vi "Weather Parse Test.vi"() -> ()   [LabVIEW 2020, in "CDM-Config.lvlib"] (continued)
,\n                    \"UGC\": [\n                        \"PKZ773\"\n                    ]\n                },\n                \"affectedZones\": [\n                    \"https://api.weather.gov/zones/forecast/PKZ773\"\n                ],\n                \"references\": [],\n                \"sent\": \"2025-12-02T16:08:00-09:00\",\n                \"effective\": \"2025-12-02T16:08:00-09:00\",\n                \"onset\": \"2025-12-03T05:00:00-09:00\",\n                \"expires\": \"2025-12-03T05:15:00-09:00\",\n                \"ends\": \"2025-12-04T05:00:00-09:00\",\n                \"status\": \"Actual\",\n                \"messageType\": \"Alert\",\n                \"category\": \"Met\",\n                \"severity\": \"Minor\",\n                \"certainty\": \"Likely\",\n                \"urgency\": \"Expected\",\n                \"event\": \"Small Craft Advisory\",\n                \"sender\": \"w-nws.webmaster@noaa.gov\",\n                \"senderName\": \"NWS Anchorage AK\",\n                \"headline\": \"Small Craft Advisory issued December 2 at 4:08PM AKST until December 4 at 5:00AM AKST by NWS Anchorage AK\",\n                \"description\": \"Coastal Waters Forecast for Southwest Alaska+Bristol Bay+The\\nAlaska Peninsula Waters and the Aleutian Islands up to 100 nm out.\\n\\nWind forecasts reflect the predominant speed and direction\\nexpected. Sea forecasts represent an average of the highest\\none-third of the combined wind wave and swell height.\\n\\n.TONIGHT...SE wind 30 kt. Seas 18 ft. Rain.\\n.WED...NE wind 25 kt. Seas 15 ft. Rain.\\n.WED NIGHT...N wind 20 kt. Seas 10 ft.\\n.THU AND THU NIGHT...NE wind 15 kt. Seas 7 ft.\\n.FRI...NE wind 25 kt. Seas 5 ft.\\n.SAT THROUGH SUN...N wind 30 kt. Seas 7 ft.\",\n                \"instruction\": null,\n                \"response\": \"Avoid\",\n                \"parameters\": {\n                    \"AWIPSidentifier\": [\n                        \"CWFALU\"\n                    ],\n                    \"WMOidentifier\": [\n                        \"FZAK52 PAFC 030108\"\n                    ],\n                    \"NWSheadline\": [\n                        \"SMALL CRAFT ADVISORY THROUGH WEDNESDAY NIGHT\"\n                    ],\n                    \"BLOCKCHANNEL\": [\n                        \"EAS\",\n                        \"NWEM\",\n                        \"CMAS\"\n                    ],\n                    \"VTEC\": [\n                        \"/O.NEW.PAFC.SC.Y.9907.251203T1400Z-251204T1400Z/\"\n                    ],\n                    \"eventEndingTime\": [\n                        \"2025-12-04T05:00:00-09:00\"\n                    ]\n                },\n                \"scope\": \"Public\",\n                \"code\": \"IPAWSv1.0\",\n                \"language\": \"en-US\",\n                \"web\": \"http://www.weather.gov\",\n                \"eventCode\": {\n                    \"SAME\": [\n                        \"NWS\"\n                    ],\n                    \"NationalWeatherService\": [\n                        \"SCY\"\n                    ]\n                }\n            }\n        },\n        {\n            \"id\": \"https://api.weather.gov/alerts/urn:oid:2.49.0.1.840.0.90d765b84bbb08e28d74a226f4e1f9e6e65de885.013.1\",\n            \"type\": \"Feature\",\n            \"geometry\": null,\n            \"properties\": {\n                \"@id\": \"https://api.weather.gov/alerts/urn:oid:2.49.0.1.840.0.90d765b84bbb08e28d74a226f4e1f9e6e65de885.013.1\",\n                \"@type\": \"wx:Alert\",\n                \"id\": \"urn:oid:2.49.0.1.840.0.90d765b84bbb08e28d74a226f4e1f9e6e65de885.013.1\",\n                \"areaDesc\": \"Cape Sarichef to Nikoski Bering Side from 15 to 85 NM\",\n                \"geocode\": {\n                    \"SAME\": [\n                        \"058772\"\n                    ],\n                    \"UGC\": [\n                        \"PKZ772\"\n                    ]\n                },\n                \"affectedZones\": [\n                    \"https://api.weather.gov/zones/forecast/PKZ772\"\n                ],\n                \"references\": [],\n                \"sent\": \"2025-12-02T16:08:00-09:00\",\n                \"effective\": \"2025-12-02T16:08:00-09:00\",\n                \"onset\": \"2025-12-03T05:00:00-09:00\",\n                \"expires\": \"2025-12-03T05:15:00-09:00\",\n                \"ends\": \"2025-12-04T05:00:00-09:00\",\n                \"status\": \"Actual\",\n                \"messageType\": \"Alert\",\n                \"category\": \"Met\",\n                \"severity\": \"Minor\",\n                \"certainty\": \"Likely\",\n                \"urgency\": \"Expected\",\n                \"event\": \"Small Craft Advisory\",\n                \"sender\": \"w-nws.webmaster@noaa.gov\",\n                \"senderName\": \"NWS Anchorage AK\",\n                \"headline\": \"Small Craft Advisory issued December 2 at 4:08PM AKST until December 4 at 5:00AM AKST by NWS Anchorage AK\",\n                \"description\": \"Coastal Waters Forecast for Southwest Alaska+Bristol Bay+The\\nAlaska Peninsula Waters and the Aleutian Islands up to 100 nm out.\\n\\nWind forecasts reflect the predominant speed and direction\\nexpected. Sea forecasts represent an average of the highest\\none-third of the combined wind wave and swell height.\\n\\n.TONIGHT...E wind 30 kt. Seas 18 ft. Rain.\\n.WED...NE wind 30 kt. Seas 15 ft. Rain.\\n.WED NIGHT...N wind 30 kt. Seas 16 ft.\\n.THU...NE wind 30 kt. Seas 14 ft.\\n.THU NIGHT...NE wind 25 kt. Seas 10 ft.\\n.FRI...NE wind 25 kt. Seas 7 ft.\\n.SAT...N wind 30 kt. Seas 15 ft.\\n.SUN...N wind 40 kt. Seas 21 ft.\",\n                \"instruction\": null,\n                \"response\": \"Avoid\",\n                \"parameters\": {\n                    \"AWIPSidentifier\": [\n                        \"CWFALU\"\n                    ],\n                    \"WMOidentifier\": [\n                        \"FZAK52 PAFC 030108\"\n                    ],\n                    \"NWSheadline\": [\n                        \"SMALL CRAFT ADVISORY THROUGH WEDNESDAY NIGHT\"\n                    ],\n                    \"BLOCKCHANNEL\": [\n                        \"EAS\",\n                        \"NWEM\",\n                        \"CMAS\"\n                    ],\n                    \"VTEC\": [\n                        \"/O.NEW.PAFC.SC.Y.9905.251203T1400Z-251204T1400Z/\"\n                    ],\n                    \"eventEndingTime\": [\n                        \"2025-12-04T05:00:00-09:00\"\n                    ]\n                },\n                \"scope\": \"Public\",\n                \"code\": \"IPAWSv1.0\",\n                \"language\": \"en-US\",\n                \"web\": \"http://www.weather.gov\",\n                \"eventCode\": {\n                    \"SAME\": [\n                        \"NWS\"\n                    ],\n                    \"NationalWeatherService\": [\n                        \"SCY\"\n                    ]\n                }\n            }\n        },\n        {\n            \"id\": \"https://api.weather.gov/alerts/urn:oid:2.49.0.1.840.0.90d765b84bbb08e28d74a226f4e1f9e6e65de885.012.1\",\n            \"type\": \"Feature\",\n            \"geometry\": null,\n            \"properties\": {\n                \"@id\": \"https://api.weather.gov/alerts/urn:oid:2.49.0.1.840.0.90d765b84bbb08e28d74a226f4e1f9e6e65de885.012.1\",\n                \"@type\": \"wx:Alert\",\n                \"id\": \"urn:oid:2.49.0.1.840.0.90d765b84bbb08e28d74a226f4e1f9e6e65de885.012.1\",\n                \"areaDesc\": \"Cape Sarichef to Nikoski Bering Side out to 15 NM\",\n                \"geocode\": {\n                    \"SAME\": [\n                        \"058770\"\n                    ],\n                    \"UGC\": [\n                        \"PKZ770\"\n                    ]\n                },\n                \"affectedZones\": [\n                    \"https://api.weather.gov/zones/forecast/PKZ770\"\n                ],\n                \"references\": [],\n                \"sent\": \"2025-12-02T16:08:00-09:00\",\n                \"effective\": \"2025-12-02T16:08:00-09:00\",\n                \"onset\": \"2025-12-03T05:00:00-09:00\",\n                \"expires\": \"2025-12-03T05:15:00-09:00\",\n                \"ends\": \"2025-12-04T05:00:00-09:00\",\n                \"status\": \"Actual\",\n                \"messageType\": \"Alert\",\n                \"category\": \"Met\",\n                \"severity\": \"Minor\",\n                \"certainty\": \"Likely\",\n                \"urgency\": \"Expected\",\n                \"event\": \"Small Craft Advisory\",\n                \"sender\": \"w-nws.webmaster@noaa.gov\",\n                \"senderName\": \"NWS Anchorage AK\",\n                \"headline\": \"Small Craft Advisory issued December 2 at 4:08PM AKST until December 4 at 5:00AM AKST by NWS Anchorage AK\",\n                \"description\": \"Coastal Waters Forecast for Southwest Alaska+Bristol Bay+The\\nAlaska Peninsula Waters and the Aleutian Islands up to 100 nm out.\\n\\nWind forecasts reflect the predominant speed and direction\\nexpected. Sea forecasts represent an average of the highest\\none-third of the combined wind wave and swell height.\\n\\n.TONIGHT...E wind 30 kt. Seas 16 ft. Rain.\\n.WED...NE wind 30 kt. Seas 13 ft. Rain.\\n.WED NIGHT...N wind 30 kt. Seas 14 ft. Rain.\\n.THU...NE wind 25 kt. Seas 13 ft.\\n.THU NIGHT...E wind 20 kt. Seas 9 ft.\\n.FRI...E wind 20 kt. Seas 6 ft.\\n.SAT...N wind 30 kt. Seas 14 ft.\\n.SUN...N wind 35 kt. Seas 18 ft.\",\n                \"instruction\": null,\n                \"response\": \"Avoid\",\n                \"parameters\": {\n                    \"AWIPSidentifier\": [\n                        \"CWFALU\"\n                    ],\n                    \"WMOidentifier\": [\n                        \"FZAK52 PAFC 030108\"\n                    ],\n                    \"NWSheadline\": [\n                        \"SMALL CRAFT ADVISORY THROUGH WEDNESDAY NIGHT\"\n                    ],\n                    \"BLOCKCHANNEL\": [\n                        \"EAS\",\n                        \"NWEM\",\n                        \"CMAS\"\n                    ],\n                    \"VTEC\": [\n                        \"/O.NEW.PAFC.SC.Y.9904.251203T1400Z-251204T1400Z/\"\n                    ],\n                    \"eventEndingTime\": [\n                        \"2025-12-04T05:00:00-09:00\"\n                    ]\n                },\n                \"scope\": \"Public\",\n                \"code\": \"IPAWSv1.0\",\n                \"language\": \"en-US\",\n                \"web\": \"http://www.weather.gov\",\n                \"eventCode\": {\n                    \"SAME\": [\n                        \"NWS\"\n                    ],\n                    \"NationalWeatherService\": [\n                        \"SCY\"\n                    ]\n                }\n            }\n        },\n        {\n            \"id\": \"https://api.weather.gov/alerts/urn:oid:2.49.0.1.840.0.90d765b84bbb08e28d74a226f4e1f9e6e65de885.018.1\",\n            \"type\": \"Feature\",\n            \"geometry\": null,\n            \"properties\": {\n                \"@id\": \"https://api.weather.gov/alerts/urn:oid:2.49.0.1.840.0.90d765b84bbb08e28d74a226f4e1f9e6e65de885.018.1\",\n                \"@type\": \"wx:Alert\",\n                \"id\": \"urn:oid:2.49.0.1.840.0.90d765b84bbb08e28d74a226f4e1f9e6e65de885.018.1\",\n                \"areaDesc\": \"Nikolski to Seguam Bering Side from 15 to 85 NM\",\n                \"geocode\": {\n                    \"SAME\": [\n                        \"058776\"\n                    ],\n                    \"UGC\": [\n                        \"PKZ776\"\n                    ]\n                },\n                \"affectedZones\": [\n                    \"https://api.weather.gov/zones/forecast/PKZ776\"\n                ],\n                \"references\": [],\n                \"sent\": \"2025-12-02T16:08:00-09:00\",\n                \"effective\": \"2025-12-02T16:08:00-09:00\",\n                \"onset\": \"2025-12-03T05:00:00-09:00\",\n                \"expires\": \"2025-12-03T05:15:00-09:00\",\n                \"ends\": \"2025-12-04T05:00:00-09:00\",\n                \"status\": \"Actual\",\n                \"messageType\": \"Alert\",\n                \"category\": \"Met\",\n                \"severity\": \"Moderate\",\n                \"certainty\": \"Likely\",\n                \"urgency\": \"Expected\",\n                \"event\": \"Gale Warning\",\n                \"sender\": \"w-nws.webmaster@noaa.gov\",\n                \"senderName\": \"NWS Anchorage AK\",\n                \"headline\": \"Gale Warning issued December 2 at 4:08PM AKST until December 4 at 5:00AM AKST by NWS Anchorage AK\",\n                \"description\": \"Coastal Waters Forecast for Southwest Alaska+Bristol Bay+The\\nAlaska Peninsula Waters and the Aleutian Islands up to 100 nm out.\\n\\nWind forecasts reflect the predominant speed and direction\\nexpected. Sea forecasts represent an average of the highest\\none-third of the combined wind wave and swell height.\\n\\n.TONIGHT...N wind 45 kt diminishing to 35 kt after midnight. Seas\\n31 ft. Rain.\\n.WED...N wind 35 kt. Seas 23 ft. Rain.\\n.WED NIGHT...N wind 35 kt. Seas 20 ft.\\n.THU...N wind 30 kt. Seas 15 ft.\\n.THU NIGHT...NE wind 20 kt. Seas 10 ft.\\n.FRI...E wind 15 kt. Seas 8 ft.\\n.SAT...N wind 30 kt. Seas 12 ft.\\n.SUN...N wind 40 kt. Seas 22 ft.\",\n                \"instruction\": null,\n                \"response\": \"Avoid\",\n                \"parameters\": {\n                    \"AWIPSidentifier\": [\n                        \"CWFALU\"\n                    ],\n                    \"WMOidentifier\": [\n                        \"FZAK52 PAFC 030108\"\n                    ],\n                    \"NWSheadline\": [\n                        \"GALE WARNING THROUGH WEDNESDAY NIGHT\"\n                    ],\n                    \"BLOCKCHANNEL\": [\n                        \"EAS\",\n                        \"NWEM\",\n                        \"CMAS\"\n                    ],\n                    \"VTEC\": [\n                        \"/O.NEW.PAFC.GL.W.9910.251203T1400Z-251204T1400Z/\"\n                    ],\n                    \"eventEndingTime\": [\n                        \"2025-12-04T05:00:00-09:00\"\n                    ]\n                },\n                \"scope\": \"Public\",\n                \"code\": \"IPAWSv1.0\",\n                \"language\": \"en-US\",\n                \"web\": \"http://www.weather.gov\",\n                \"eventCode\": {\n                    \"SAME\": [\n                        \"NWS\"\n                    ],\n                    \"NationalWeatherService\": [\n                        \"GLW\"\n                    ]\n                }\n            }\n        },\n        {\n            \"id\": \"https://api.weather.gov/alerts/urn:oid:2.49.0.1.840.0.90d765b84bbb08e28d74a226f4e1f9e6e65de885.004.1\",\n            \"type\": \"Feature\",\n            \"geometry\": null,\n            \"properties\": {\n                \"@id\": \"https://api.weather.gov/alerts/urn:oid:2.49.0.1.840.0.90d765b84bbb08e28d74a226f4e1f9e6e65de885.004.1\",\n                \"@type\": \"wx:Alert\",\n                \"id\": \"urn:oid:2.49.0.1.840.0.90d765b84bbb08e28d74a226f4e1f9e6e65de885.004.1\",\n                \"areaDesc\": \"Castle Cape to Cape Tolstoi out to 15 NM\",\n                \"geocode\": {\n                    \"SAME\": [\n                        \"058752\"\n                    ],\n                    \"UGC\": [\n                        \"PKZ752\"\n                    ]\n                },\n                \"affectedZones\": [\n                    \"https://api.weather.gov/zones/forecast/PKZ752\"\n                ],\n                \"references\": [],\n                \"sent\": \"2025-12-02T16:08:00-09:00\",\n                \"effective\": \"2025-12-02T16:08:00-09:00\",\n                \"onset\": \"2025-12-03T05:00:00-09:00\",\n                \"expires\": \"2025-12-03T05:15:00-09:00\",\n                \"ends\": \"2025-12-04T05:00:00-09:00\",\n                \"status\": \"Actual\",\n                \"messageType\": \"Alert\",\n                \"category\": \"Met\",\n                \"severity\": \"Minor\",\n                \"certainty\": \"Likely\",\n                \"urgency\": \"Expected\",\n                \"event\": \"Small Craft Advisory\",\n                \"sender\": \"w-nws.webmaster@noaa.gov\",\n                \"senderName\": \"NWS Anchorage AK\",\n                \"headline\": \"Small Craft Advisory issued December 2 at 4:08PM AKST until December 4 at 5:00AM AKST by NWS Anchorage AK\",\n                \"description\": \"Coastal Waters Forecast for Southwest Alaska+Bristol Bay+The\\nAlaska Peninsula Waters and the Aleutian Islands up to 100 nm out.\\n\\nWind forecasts reflect the predominant speed and direction\\nexpected. Sea forecasts represent an average of the highest\\none-third of the combined wind wave and swell height.\\n\\n.TONIGHT...SE wind 25 kt. Seas 13 ft. Rain.\\n.WED...SE wind 20 kt. Seas 10 ft. Rain.\\n.WED NIGHT...SE wind 20 kt. Seas 10 ft. Rain.\\n.THU...E wind 20 kt. Seas 8 ft.\\n.THU NIGHT...NE wind 25 kt. Seas 8 ft.\\n.FRI...N wind 20 kt. Seas 8 ft.\\n.SAT...NW wind 35 kt. Seas 5 ft.\\n.SUN...N wind 20 kt. Seas 2 ft.\",\n                \"instruction\": null,\n                \"response\": \"Avoid\",\n                \"parameters\": {\n                    \"AWIPSidentifier\": [\n                        \"CWFALU\"\n                    ],\n                    \"WMOidentifier\": [\n                        \"FZAK52 PAFC 030108\"\n                    ],\n                    \"NWSheadline\": [\n                        \"SMALL CRAFT ADVISORY THROUGH WEDNESDAY NIGHT\"\n                    ],\n                    \"BLOCKCHANNEL\": [\n                        \"EAS\",\n                        \"NWEM\",\n                        \"CMAS\"\n                    ],\n                    \"VTEC\": [\n                        \"/O.NEW.PAFC.SC.Y.9896.251203T1400Z-251204T1400Z/\"\n                    ],\n                    \"eventEndingTime\": [\n                        \"2025-12-04T05:00:00-09:00\"\n                    ]\n                },\n                \"scope\": \"Public\",\n                \"code\": \"IPAWSv1.0\",\n                \"language\": \"en-US\",\n                \"web\": \"http://www.weather.gov\",\n                \"eventCode\": {\n                    \"SAME\": [\n                        \"NWS\"\n                    ],\n                    \"NationalWeatherService\": [\n                        \"SCY\"\n                    ]\n                }\n            }\n        },\n        {\n            \"id\": \"https://api.weather.gov/alerts/urn:oid:2.49.0.1.840.0.90d765b84bbb08e28d74a226f4e1f9e6e65de885.005.1\",\n            \"type\": \"Feature\",\n            \"geometry\": null,\n            \"properties\": {\n                \"@id\": \"https://api.weather.gov/alerts/urn:oid:2.49.0.1.840.0.90d765b84bbb08e28d74a226f4e1f9e6e65de885.005.1\",\n                \"@type\": \"wx:Alert\",\n                \"id\": \"urn:oid:2.49.0.1.840.0.90d765b84bbb08e28d74a226f4e1f9e6e65de885.005.1\",\n                \"areaDesc\": \"Castle Cape to Cape Tolstoi from 15 to 100 NM\",\n                \"geocode\": {\n                    \"SAME\": [\n                        \"058753\"\n                    ],\n                    \"UGC\": [\n                        \"PKZ753\"\n                    ]\n                },\n                \"affectedZones\": [\n                    \"https://api.weather.gov/zones/forecast/PKZ753\"\n                ],\n                \"references\": [],\n                \"sent\": \"2025-12-02T16:08:00-09:00\",\n                \"effective\": \"2025-12-02T16:08:00-09:00\",\n                \"onset\": \"2025-12-03T05:00:00-09:00\",\n                \"expires\": \"2025-12-03T05:15:00-09:00\",\n                \"ends\": \"2025-12-04T05:00:00-09:00\",\n                \"status\": \"Actual\",\n                \"messageType\": \"Alert\",\n                \"category\": \"Met\",\n                \"severity\": \"Minor\",\n                \"certainty\": \"Likely\",\n                \"urgency\": \"Expected\",\n                \"event\": \"Small Craft Advisory\",\n                \"sender\": \"w-nws.webmaster@noaa.gov\",\n                \"senderName\": \"NWS Anchorage AK\",\n                \"headline\": \"Small Craft Advisory issued December 2 at 4:08PM AKST until December 4 at 5:00AM AKST by NWS Anchorage AK\",\n                \"description\": \"Coastal Waters Forecast for Southwest Alaska+Bristol Bay+The\\nAlaska Peninsula Waters and the Aleutian Islands up to 100 nm out.\\n\\nWind forecasts reflect the predominant speed and direction\\nexpected. Sea forecasts represent an average of the highest\\none-third of the combined wind wave and swell height.\\n\\n.TONIGHT...SE wind 30 kt. Seas 19 ft.\\n.WED...S wind 25 kt. Seas 17 ft. Rain.\\n.WED NIGHT...S wind 20 kt. Seas 16 ft. Rain.\\n.THU...E wind 20 kt. Seas 12 ft.\\n.THU NIGHT...NE wind 30 kt. Seas 9 ft.\\n.FRI...NW wind 20 kt. Seas 9 ft.\\n.SAT...NW wind 35 kt. Seas 13 ft.\\n.SUN...N wind 25 kt. Seas 11 ft.\",\n                \"instruction\": null,\n                \"response\": \"Avoid\",\n                \"parameters\": {\n                    \"AWIPSidentifier\": [\n                        \"CWFALU\"\n                    ],\n                    \"WMOidentifier\": [\n                        \"FZAK52 PAFC 030108\"\n                    ],\n                    \"NWSheadline\": [\n                        \"SMALL CRAFT ADVISORY THROUGH WEDNESDAY NIGHT\"\n                    ],\n                    \"BLOCKCHANNEL\": [\n                        \"EAS\",\n                        \"NWEM\",\n                        \"CMAS\"\n                    ],\n                    \"VTEC\": [\n                        \"/O.NEW.PAFC.SC.Y.9897.251203T1400Z-251204T1400Z/\"\n                    ],\n                    \"eventEndingTime\": [\n                        \"2025-12-04T05:00:00-09:00\"\n                    ]\n                },\n                \"scope\": \"Public\",\n                \"code\": \"IPAWSv1.0\",\n                \"language\": \"en-US\",\n                \"web\": \"http://www.weather.gov\",\n                \"eventCode\": {\n                    \"SAME\": [\n                        \"NWS\"\n                    ],\n                    \"NationalWeatherService\": [\n                        \"SCY\"\n                    ]\n                }\n            }\n        },\n        {\n            \"id\": \"https://api.weather.gov/alerts/urn:oid:2.49.0.1.840.0.90d765b84bbb08e28d74a226f4e1f9e6e65de885.023.1\",\n            \"type\": \"Feature\",\n            \"geometry\": null,\n            \"properties\": {\n                \"@id\": \"https://api.weather.gov/alerts/urn:oid:2.49.0.1.840.0.90d765b84bbb08e28d74a226f4e1f9e6e65de885.023.1\",\n                \"@type\": \"wx:Alert\",\n                \"id\": \"urn:oid:2.49.0.1.840.0.90d765b84bbb08e28d74a226f4e1f9e6e65de885.023.1\",\n                \"areaDesc\": \"Seguam to Adak Pacific Side out to 15 NM\",\n                \"geocode\": {\n                    \"SAME\": [\n                        \"058782\"\n                    ],\n                    \"UGC\": [\n                        \"PKZ782\"\n                    ]\n                },\n                \"affectedZones\": [\n                    \"https://api.weather.gov/zones/forecast/PKZ782\"\n                ],\n                \"references\": [],\n                \"sent\": \"2025-12-02T16:08:00-09:00\",\n                \"effective\": \"2025-12-02T16:08:00-09:00\",\n                \"onset\": \"2025-12-02T16:00:00-09:00\",\n                \"expires\": \"2025-12-03T05:15:00-09:00\",\n                \"ends\": \"2025-12-03T17:00:00-09:00\",\n                \"status\": \"Actual\",\n                \"messageType\": \"Alert\",\n                \"category\": \"Met\",\n                \"severity\": \"Moderate\",\n                \"certainty\": \"Likely\",\n                \"urgency\": \"Expected\",\n                \"event\": \"Gale Warning\",\n                \"sender\": \"w-nws.webmaster@noaa.gov\",\n                \"senderName\": \"NWS Anchorage AK\",\n                \"headline\": \"Gale Warning issued December 2 at 4:08PM AKST until December 3 at 5:00PM AKST by NWS Anchorage AK\",\n                \"description\": \"Coastal Waters Forecast for Southwest Alaska+Bristol Bay+The\\nAlaska Peninsula Waters and the Aleutian Islands up to 100 nm out.\\n\\nWind forecasts reflect the predominant speed and direction\\nexpected. Sea forecasts represent an average of the highest\\none-third of the combined wind wave and swell height.\\n\\n.TONIGHT...N wind 45 kt. Seas 15 ft. Rain.\\n.WED...N wind 35 kt. Seas 14 ft. Rain.\\n.WED NIGHT...N wind 30 kt. Seas 11 ft.\\n.THU...N wind 30 kt. Seas 8 ft.\\n.THU NIGHT...NE wind 15 kt. Seas 5 ft.\\n.FRI...NE wind 15 kt. Seas 10 ft.\\n.SAT...NE wind 25 kt. Seas 10 ft.\\n.SUN...N wind 35 kt. Seas 12 ft.\",\n                \"instruction\": null,\n                \"response\": \"Avoid\",\n                \"parameters\": {\n                    \"AWIPSidentifier\": [\n                        \"CWFALU\"\n                    ],\n                    \"WMOidentifier\": [\n                        \"FZAK52 PAFC 030108\"\n                    ],\n                    \"NWSheadline\": [\n                        \"GALE WARNING THROUGH WEDNESDAY\"\n                    ],\n                    \"BLOCKCHANNEL\": [\n                        \"EAS\",\n                        \"NWEM\",\n                        \"CMAS\"\n                    ],\n                    \"VTEC\": [\n                        \"/O.NEW.PAFC.GL.W.9915.251203T0100Z-251204T0200Z/\"\n                    ],\n                    \"eventEndingTime\": [\n                        \"2025-12-03T17:00:00-09:00\"\n                    ]\n                },\n                \"scope\": \"Public\",\n                \"code\": \"IPAWSv1.0\",\n                \"language\": \"en-US\",\n                \"web\": \"http://www.weather.gov\",\n                \"eventCode\": {\n                    \"SAME\": [\n                        \"NWS\"\n                    ],\n                    \"NationalWeatherService\": [\n                        \"GLW\"\n                    ]\n                }\n            }\n        },\n        {\n            \"id\": \"https://api.weather.gov/alerts/urn:oid:2.49.0.1.840.0.90d765b84bbb08e28d74a226f4e1f9e6e65de885.026.1\",\n            \"type\": \"Feature\",\n            \"geometry\": null,\n            \"properties\": {\n                \"@id\": \"https://api.weather.gov/alerts/urn:oid:2.49.0.1.840.0.90d765b84bbb08e28d74a226f4e1f9e6e65de885.026.1\",\n                \"@type\": \"wx:Alert\",\n                \"id\": \"urn:oid:2.49.0.1.840.0.90d765b84bbb08e28d74a226f4e1f9e6e65de885.026.1\",\n                \"areaDesc\": \"Adak to Kiska Pacific Side\",\n                \"geocode\": {\n                    \"SAME\": [\n                        \"058785\"\n                    ],\n                    \"UGC\": [\n                        \"PKZ785\"\n                    ]\n                },\n                \"affectedZones\": [\n                    \"https://api.weather.gov/zones/forecast/PKZ785\"\n                ],\n                \"references\": [],\n                \"sent\": \"2025-12-02T16:08:00-09:00\",\n                \"effective\": \"2025-12-02T16:08:00-09:00\",\n                \"onset\": \"2025-12-02T16:00:00-09:00\",\n                \"expires\": \"2025-12-03T05:15:00-09:00\",\n                \"ends\": \"2025-12-03T17:00:00-09:00\",\n                \"status\": \"Actual\",\n                \"messageType\": \"Alert\",\n                \"category\": \"Met\",\n                \"severity\": \"Moderate\",\n                \"certainty\": \"Likely\",\n                \"urgency\": \"Expected\",\n                \"event\": \"Gale Warning\",\n                \"sender\": \"w-nws.webmaster@noaa.gov\",\n                \"senderName\": \"NWS Anchorage AK\",\n                \"headline\": \"Gale Warning issued December 2 at 4:08PM AKST until December 3 at 5:00PM AKST by NWS Anchorage AK\",\n                \"description\": \"Coastal Waters Forecast for Southwest Alaska+Bristol Bay+The\\nAlaska Peninsula Waters and the Aleutian Islands up to 100 nm out.\\n\\nWind forecasts reflect the predominant speed and direction\\nexpected. Sea forecasts represent an average of the highest\\none-third of the combined wind wave and swell height.\\n\\n.TONIGHT...N wind 40 kt. Seas 21 ft.\\n.WED...N wind 40 kt. Seas 20 ft.\\n.WED NIGHT...N wind 30 kt. Seas 15 ft.\\n.THU...E wind 25 kt. Seas 10 ft.\\n.THU NIGHT...SE wind 30 kt. Seas 11 ft.\\n.FRI...NW wind 30 kt. Seas 15 ft.\\n.SAT...NE wind 20 kt. Seas 12 ft.\\n.SUN...NE wind 30 kt. Seas 12 ft.\",\n                \"instruction\": null,\n                \"response\": \"Avoid\",\n                \"parameters\": {\n                    \"AWIPSidentifier\": [\n                        \"CWFALU\"\n                    ],\n                    \"WMOidentifier\": [\n                        \"FZAK52 PAFC 030108\"\n                    ],\n                    \"NWSheadline\": [\n                        \"GALE WARNING THROUGH WEDNESDAY\"\n                    ],\n                    \"BLOCKCHANNEL\": [\n                        \"EAS\",\n                        \"NWEM\",\n                        \"CMAS\"\n                    ],\n                    \"VTEC\": [\n                        \"/O.NEW.PAFC.GL.W.9918.251203T0100Z-251204T0200Z/\"\n                    ],\n                    \"eventEndingTime\": [\n                        \"2025-12-03T17:00:00-09:00\"\n                    ]\n                },\n                \"scope\": \"Public\",\n                \"code\": \"IPAWSv1.0\",\n                \"language\": \"en-US\",\n                \"web\": \"http://www.weather.gov\",\n                \"eventCode\": {\n                    \"SAME\": [\n                        \"NWS\"\n                    ],\n                    \"NationalWeatherService\": [\n                        \"GLW\"\n                    ]\n                }\n            }\n        },\n        {\n            \"id\": \"https://api.weather.gov/alerts/urn:oid:2.49.0.1.840.0.90d765b84bbb08e28d74a226f4e1f9e6e65de885.021.1\",\n            \"type\": \"Feature\",\n            \"geometry\": null,\n            \"properties\": {\n                \"@id\": \"https://api.weather.gov/alerts/urn:oid:2.49.0.1.840.0.90d765b84bbb08e28d74a226f4e1f9e6e65de885.021.1\",\n                \"@type\": \"wx:Alert\",\n                \"id\": \"urn:oid:2.49.0.1.840.0.90d765b84bbb08e28d74a226f4e1f9e6e65de885.021.1\",\n                \"areaDesc\": \"Seguam to Adak Bering Side out to 15 NM\",\n                \"geocode\": {\n                    \"SAME\": [\n                        \"058780\"\n                    ],\n                    \"UGC\": [\n                        \"PKZ780\"\n                    ]\n                },\n                \"affectedZones\": [\n                    \"https://api.weather.gov/zones/forecast/PKZ780\"\n                ],\n                \"references\": [],\n                \"sent\": \"2025-12-02T16:08:00-09:00\",\n                \"effective\": \"2025-12-02T16:08:00-09:00\",\n                \"onset\": \"2025-12-02T16:00:00-09:00\",\n                \"expires\": \"2025-12-03T05:15:00-09:00\",\n                \"ends\": \"2025-12-03T17:00:00-09:00\",\n                \"status\": \"Actual\",\n                \"messageType\": \"Alert\",\n                \"category\": \"Met\",\n                \"severity\": \"Moderate\",\n                \"certainty\": \"Likely\",\n                \"urgency\": \"Expected\",\n                \"event\": \"Gale Warning\",\n                \"sender\": \"w-nws.webmaster@noaa.gov\",\n                \"senderName\": \"NWS Anchorage AK\",\n                \"headline\": \"Gale Warning issued December 2 at 4:08PM AKST until December 3 at 5:00PM AKST by NWS Anchorage AK\",\n                \"description\": \"Coastal Waters Forecast for Southwest Alaska+Bristol Bay+The\\nAlaska Peninsula Waters and the Aleutian Islands up to 100 nm out.\\n\\nWind forecasts reflect the predominant speed and direction\\nexpected. Sea forecasts represent an average of the highest\\none-third of the combined wind wave and swell height.\\n\\n.TONIGHT...N wind 45 kt. Seas 30 ft. Rain.\\n.WED...N wind 40 kt. Seas 27 ft. Rain.\\n.WED NIGHT...N wind 30 kt. Seas 21 ft.\\n.THU...N wind 30 kt. Seas 15 ft.\\n.THU NIGHT...NE wind 15 kt. Seas 10 ft.\\n.FRI...Variable wind 10 kt. Seas 7 ft.\\n.SAT...NE wind 25 kt. Seas 8 ft.\\n.SUN...NE wind 35 kt. Seas 20 ft.\",\n                \"instruction\": null,\n                \"response\": \"Avoid\",\n                \"parameters\": {\n                    \"AWIPSidentifier\": [\n                        \"CWFALU\"\n                    ],\n                    \"WMOidentifier\": [\n                        \"FZAK52 PAFC 030108\"\n                    ],\n                    \"NWSheadline\": [\n                        \"GALE WARNING THROUGH WEDNESDAY\"\n                    ],\n                    \"BLOCKCHANNEL\": [\n                        \"EAS\",\n                        \"NWEM\",\n                        \"CMAS\"\n                    ],\n                    \"VTEC\": [\n                        \"/O.NEW.PAFC.GL.W.9913.251203T0100Z-251204T0200Z/\"\n                    ],\n                    \"eventEndingTime\": [\n                        \"2025-12-03T17:00:00-09:00\"\n                    ]\n                },\n                \"scope\": \"Public\",\n                \"code\": \"IPAWSv1.0\",\n                \"language\": \"en-US\",\n                \"web\": \"http://www.weather.gov\",\n                \"eventCode\": {\n                    \"SAME\": [\n                        \"NWS\"\n                    ],\n                    \"NationalWeatherService\": [\n                        \"GLW\"\n                    ]\n                }\n            }\n        },\n        {\n            \"id\": \"https://api.weather.gov/alerts/urn:oid:2.49.0.1.840.0.90d765b84bbb08e28d74a226f4e1f9e6e65de885.032.1\",\n            \"type\": \"Feature\",\n            \"geometry\": null,\n            \"properties\": {\n                \"@id\": \"https://api.weather.gov/alerts/urn:oid:2.49.0.1.840.0.90d765b84bbb08e28d74a226f4e1f9e6e65de885.032.1\",\n                \"@type\": \"wx:Alert\",\n                \"id\": \"urn:oid:2.49.0.1.840.0.90d765b84bbb08e28d74a226f4e1f9e6e65de885.032.1\",\n                \"areaDesc\": \"Bristol Bay from Cape Chichagof to Cape Pierce out to 15 NM\",\n                \"geocode\": {\n                    \"SAME\": [\n                        \"058762\"\n                    ],\n                    \"UGC\": [\n                        \"PKZ762\"\n                    ]\n                },\n                \"affectedZones\": [\n                    \"https://api.weather.gov/zones/forecast/PKZ762\"\n                ],\n                \"references\": [],\n                \"sent\": \"2025-12-02T16:08:00-09:00\",\n                \"effective\": \"2025-12-02T16:08:00-09:00\",\n                \"onset\": \"2025-12-03T05:00:00-09:00\",\n                \"expires\": \"2025-12-03T05:15:00-09:00\",\n                \"ends\": \"2025-12-04T05:00:00-09:00\",\n                \"status\": \"Actual\",\n                \"messageType\": \"Alert\",\n                \"category\": \"Met\",\n                \"severity\": \"Minor\",\n                \"certainty\": \"Likely\",\n                \"urgency\": \"Expected\",\n                \"event\": \"Small Craft Advisory\",\n                \"sender\": \"w-nws.webmaster@noaa.gov\",\n                \"senderName\": \"NWS Anchorage AK\",\n                \"headline\": \"Small Craft Advisory issued December 2 at 4:08PM AKST until December 4 at 5:00AM AKST by NWS Anchorage AK\",\n                \"description\": \"Coastal Waters Forecast for Southwest Alaska+Bristol Bay+The\\nAlaska Peninsula Waters and the Aleutian Islands up to 100 nm out.\\n\\nWind forecasts reflect the predominant speed and direction\\nexpected. Sea forecasts represent an average of the highest\\none-third of the combined wind wave and swell height.\\n\\n.TONIGHT...E wind 25 kt. Seas 4 ft. Areas of fog. Rain.\\n.WED...NE wind 25 kt. Seas 4 ft. Rain.\\n.WED NIGHT...NE wind 25 kt. Seas 4 ft. Rain.\\n.THU AND THU NIGHT...NE wind 25 kt. Seas 4 ft.\\n.FRI...N wind 30 kt. Seas 3 ft.\\n.SAT...N wind 35 kt. Seas 5 ft.\\n.SUN...N wind 30 kt. Seas 3 ft.\",\n                \"instruction\": null,\n                \"response\": \"Avoid\",\n                \"parameters\": {\n                    \"AWIPSidentifier\": [\n                        \"CWFALU\"\n                    ],\n                    \"WMOidentifier\": [\n                        \"FZAK52 PAFC 030108\"\n                    ],\n                    \"NWSheadline\": [\n                        \"SMALL CRAFT ADVISORY THROUGH WEDNESDAY NIGHT\"\n                    ],\n                    \"BLOCKCHANNEL\": [\n                        \"EAS\",\n                        \"NWEM\",\n                        \"CMAS\"\n                    ],\n                    \"VTEC\": [\n                        \"/O.NEW.PAFC.SC.Y.9924.251203T1400Z-251204T1400Z/\"\n                    ],\n                    \"eventEndingTime\": [\n                        \"2025-12-04T05:00:00-09:00\"\n                    ]\n                },\n                \"scope\": \"Public\",\n                \"code\": \"IPAWSv1.0\",\n                \"language\": \"en-US\",\n                \"web\": \"http://www.weather.gov\",\n                \"eventCode\": {\n                    \"SAME\": [\n                        \"NWS\"\n                    ],\n                    \"NationalWeatherService\": [\n                        \"SCY\"\n                    ]\n                }\n            }\n        },\n        {\n            \"id\": \"https://api.weather.gov/alerts/urn:oid:2.49.0.1.840.0.90d765b84bbb08e28d74a226f4e1f9e6e65de885.031.1\",\n            \"type\": \"Feature\",\n            \"geometry\": null,\n            \"properties\": {\n                \"@id\": \"https://api.weather.gov/alerts/urn:oid:2.49.0.1.840.0.90d765b84bbb08e28d74a226f4e1f9e6e65de885.031.1\",\n                \"@type\": \"wx:Alert\",\n                \"id\": \"urn:oid:2.49.0.1.840.0.90d765b84bbb08e28d74a226f4e1f9e6e65de885.031.1\",\n                \"areaDesc\": \"Bristol Bay from Port Heiden to Cape Chichagof out to 15 NM\",\n                \"geocode\": {\n                    \"SAME\": [\n                        \"058761\"\n                    ],\n                    \"UGC\": [\n                        \"PKZ761\"\n                    ]\n                },\n                \"affectedZones\": [\n                    \"https://api.weather.gov/zones/forecast/PKZ761\"\n                ],\n                \"references\": [],\n                \"sent\": \"2025-12-02T16:08:00-09:00\",\n                \"effective\": \"2025-12-02T16:08:00-09:00\",\n                \"onset\": \"2025-12-02T16:00:00-09:00\",\n                \"expires\": \"2025-12-03T05:15:00-09:00\",\n                \"ends\": \"2025-12-03T17:00:00-09:00\",\n                \"status\": \"Actual\",\n                \"messageType\": \"Alert\",\n                \"category\": \"Met\",\n                \"severity\": \"Minor\",\n                \"certainty\": \"Likely\",\n                \"urgency\": \"Expected\",\n                \"event\": \"Small Craft Advisory\",\n                \"sender\": \"w-nws.webmaster@noaa.gov\",\n                \"senderName\": \"NWS Anchorage AK\",\n                \"headline\": \"Small Craft Advisory issued December 2 at 4:08PM AKST until December 3 at 5:00PM AKST by NWS Anchorage AK\",\n                \"description\": \"Coastal Waters Forecast for Southwest Alaska+Bristol Bay+The\\nAlaska Peninsula Waters and the Aleutian Islands up to 100 nm out.\\n\\nWind forecasts reflect the predominant speed and direction\\nexpected. Sea forecasts represent an average of the highest\\none-third of the combined wind wave and swell height.\\n\\n.TONIGHT...SE wind 25 kt. Seas 4 ft.\\n.WED...E wind 25 kt. Seas 4 ft.\\n.WED NIGHT...E wind 20 kt. Seas 2 ft.\\n.THU...E wind 20 kt. Seas 2 ft.\\n.THU NIGHT...NE wind 25 kt. Seas 5 ft.\\n.FRI...N wind 30 kt. Seas 6 ft.\\n.SAT...N wind 35 kt. Seas 8 ft.\\n.SUN...NE wind 30 kt. Seas 6 ft.\",\n                \"instruction\": null,\n                \"response\": \"Avoid\",\n                \"parameters\": {\n                    \"AWIPSidentifier\": [\n                        \"CWFALU\"\n                    ],\n                    \"WMOidentifier\": [\n                        \"FZAK52 PAFC 030108\"\n                    ],\n                    \"NWSheadline\": [\n                        \"SMALL CRAFT ADVISORY THROUGH WEDNESDAY\"\n                    ],\n                    \"BLOCKCHANNEL\": [\n                        \"EAS\",\n                        \"NWEM\",\n                        \"CMAS\"\n                    ],\n                    \"VTEC\": [\n                        \"/O.NEW.PAFC.SC.Y.9923.251203T0100Z-251204T0200Z/\"\n                    ],\n                    \"eventEndingTime\": [\n                        \"2025-12-03T17:00:00-09:00\"\n                    ]\n                },\n                \"scope\": \"Public\",\n                \"code\": \"IPAWSv1.0\",\n                \"language\": \"en-US\",\n                \"web\": \"http://www.weather.gov\",\n                \"eventCode\": {\n                    \"SAME\": [\n                        \"NWS\"\n                    ],\n                    \"NationalWeatherService\": [\n                        \"SCY\"\n                    ]\n                }\n            }\n        },\n        {\n            \"id\": \"https://api.weather.gov/alerts/urn:oid:2.49.0.1.840.0.90d765b84bbb08e28d74a226f4e1f9e6e65de885.035.1\",\n            \"type\": \"Feature\",\n            \"geometry\": null,\n            \"properties\": {\n                \"@id\": \"https://api.weather.gov/alerts/urn:oid:2.49.0.1.840.0.90d765b84bbb08e28d74a226f4e1f9e6e65de885.035.1\",\n                \"@type\": \"wx:Alert\",\n                \"id\": \"urn:oid:2.49.0.1.840.0.90d765b84bbb08e28d74a226f4e1f9e6e65de885.035.1\",\n                \"areaDesc\": \"North and West of Nunivak Island\",\n                \"geocode\": {\n                    \"SAME\": [\n                        \"058765\"\n                    ],\n                    \"UGC\": [\n                        \"PKZ765\"\n                    ]\n                },\n                \"affectedZones\": [\n                    \"https://api.weather.gov/zones/forecast/PKZ765\"\n                ],\n                \"references\": [],\n                \"sent\": \"2025-12-02T16:08:00-09:00\",\n                \"effective\": \"2025-12-02T16:08:00-09:00\",\n                \"onset\": \"2025-12-03T05:00:00-09:00\",\n                \"expires\": \"2025-12-03T05:15:00-09:00\",\n                \"ends\": \"2025-12-04T05:00:00-09:00\",\n                \"status\": \"Actual\",\n                \"messageType\": \"Alert\",\n                \"category\": \"Met\",\n                \"severity\": \"Moderate\",\n                \"certainty\": \"Likely\",\n                \"urgency\": \"Expected\",\n                \"event\": \"Gale Warning\",\n                \"sender\": \"w-nws.webmaster@noaa.gov\",\n                \"senderName\": \"NWS Anchorage AK\",\n                \"headline\": \"Gale Warning issued December 2 at 4:08PM AKST until December 4 at 5:00AM AKST by NWS Anchorage AK\",\n                \"description\": \"Coastal Waters Forecast for Southwest Alaska+Bristol Bay+The\\nAlaska Peninsula Waters and the Aleutian Islands up to 100 nm out.\\n\\nWind forecasts reflect the predominant speed and direction\\nexpected. Sea forecasts represent an average of the highest\\none-third of the combined wind wave and swell height.\\n\\n.TONIGHT...NE wind 45 kt. Seas 16 ft. Snow. Freezing spray.\\n.WED...NE wind 40 kt. Seas 14 ft. Snow. Freezing spray.\\n.WED NIGHT...NE wind 35 kt. Seas 11 ft. Freezing spray.\\n.THU...NE wind 30 kt. Seas 8 ft.\\n.THU NIGHT...NE wind 25 kt. Seas 6 ft.\\n.FRI...NE wind 25 kt. Seas 5 ft.\\n.SAT THROUGH SUN...NE wind 40 kt. Seas 15 ft.\",\n                \"instruction\": null,\n                \"response\": \"Avoid\",\n                \"parameters\": {\n                    \"AWIPSidentifier\": [\n                        \"CWFALU\"\n                    ],\n                    \"WMOidentifier\": [\n                        \"FZAK52 PAFC 030108\"\n                    ],\n                    \"NWSheadline\": [\n                        \"GALE WARNING THROUGH WEDNESDAY NIGHT\"\n                    ],\n                    \"BLOCKCHANNEL\": [\n                        \"EAS\",\n                        \"NWEM\",\n                        \"CMAS\"\n                    ],\n                    \"VTEC\": [\n                        \"/O.NEW.PAFC.GL.W.9927.251203T1400Z-251204T1400Z/\"\n                    ],\n                    \"eventEndingTime\": [\n                        \"2025-12-04T05:00:00-09:00\"\n                    ]\n                },\n                \"scope\": \"Public\",\n                \"code\": \"IPAWSv1.0\",\n                \"language\": \"en-US\",\n                \"web\": \"http://www.weather.gov\",\n                \"eventCode\": {\n                    \"SAME\": [\n                        \"NWS\"\n                    ],\n                    \"NationalWeatherService\": [\n                        \"GLW\"\n                    ]\n                }\n            }\n        },\n        {\n            \"id\": \"https://api.weather.gov/alerts/urn:oid:2.49.0.1.840.0.2a1d2401ea80a7d4927e142ee65572f17443d0ca.005.1\",\n            \"type\": \"Feature\",\n            \"geometry\": null,\n            \"properties\": {\n                \"@id\": \"https://api.weather.gov/alerts/urn:oid:2.49.0.1.840.0.2a1d2401ea80a7d4927e142ee65572f17443d0ca.005.1\",\n                \"@type\": \"wx:Alert\",\n                \"id\": \"urn:oid:2.49.0.1.840.0.2a1d2401ea80a7d4927e142ee65572f17443d0ca.005.1\",\n                \"areaDesc\": \"Bering Sea Offshore East of 171W\",\n                \"geocode\": {\n                    \"SAME\": [\n                        \"058414\"\n                    ],\n                    \"UGC\": [\n                        \"PKZ414\"\n                    ]\n                },\n                \"affectedZones\": [\n                    \"https://api.weather.gov/zones/forecast/PKZ414\"\n                ],\n                \"references\": [],\n                \"sent\": \"2025-12-02T16:03:00-09:00\",\n                \"effective\": \"2025-12-02T16:03:00-09:00\",\n                \"onset\": \"2025-12-03T05:00:00-09:00\",\n                \"expires\": \"2025-12-03T06:15:00-09:00\",\n                \"ends\": \"2025-12-04T05:00:00-09:00\",\n                \"status\": \"Actual\",\n                \"messageType\": \"Alert\",\n                \"category\": \"Met\",\n                \"severity\": \"Moderate\",\n                \"certainty\": \"Likely\",\n                \"urgency\": \"Expected\",\n                \"event\": \"Gale Warning\",\n                \"sender\": \"w-nws.webmaster@noaa.gov\",\n                \"senderName\": \"NWS Anchorage AK\",\n                \"headline\": \"Gale Warning issued December 2 at 4:03PM AKST until December 4 at 5:00AM AKST by NWS Anchorage AK\",\n                \"description\": \"Offshore Waters Forecast for the Bering Sea\\n\\nWind forecasts reflect the predominant speed and direction\\nexpected. Sea forecasts represent an average of the highest\\none-third of the combined wind wave and swell height.\\n\\n.TONIGHT...NE wind 30 to 45 kt. Seas 12 to 20 ft. Rain and snow.\\n.WED...NE wind 25 to 40 kt. Seas 9 to 17 ft. Rain and snow.\\n.WED NIGHT...NE wind 25 to 35 kt. Seas 9 to 16 ft. Rain.\\n.THU...NE wind 30 kt. Seas 9 to 14 ft.\\n.THU NIGHT...NE wind 20 to 30 kt. Seas 7 to 11 ft.\\n.FRI...NE wind 10 to 25 kt. Seas 5 to 8 ft.\\n.SAT...N wind 25 to 40 kt. Seas 9 to 14 ft.\\n.SUN...NE wind 30 to 40 kt. Seas 14 to 21 ft.\",\n                \"instruction\": null,\n                \"response\": \"Avoid\",\n                \"parameters\": {\n                    \"AWIPSidentifier\": [\n                        \"OFFALU\"\n                    ],\n                    \"WMOidentifier\": [\n                        \"FZAK62 PAFC 030103\"\n                    ],\n                    \"NWSheadline\": [\n                        \"GALE WARNING THROUGH WEDNESDAY NIGHT\"\n                    ],\n                    \"BLOCKCHANNEL\": [\n                        \"EAS\",\n                        \"NWEM\",\n                        \"CMAS\"\n                    ],\n                    \"VTEC\": [\n                        \"/O.NEW.PAFC.GL.W.6406.251203T1400Z-251204T1400Z/\"\n                    ],\n                    \"eventEndingTime\": [\n                        \"2025-12-04T05:00:00-09:00\"\n                    ]\n                },\n                \"scope\": \"Public\",\n                \"code\": \"IPAWSv1.0\",\n                \"language\": \"en-US\",\n                \"web\": \"http://www.weather.gov\",\n                \"eventCode\": {\n                    \"SAME\": [\n                        \"NWS\"\n                    ],\n                    \"NationalWeatherService\": [\n                        \"GLW\"\n                    ]\n                }\n            }\n        },\n        {\n            \"id\": \"https://api.weather.gov/alerts/urn:oid:2.49.0.1.840.0.52fef07b0c3a98d88109cd1837a99c72cb982c5b.011.2\",\n            \"type\": \"Feature\",\n            \"geometry\": null,\n            \"properties\": {\n                \"@id\": \"https://api.weather.gov/alerts/urn:oid:2.49.0.1.840.0.52fef07b0c3a98d88109cd1837a99c72cb982c5b.011.2\",\n                \"@type\": \"wx:Alert\",\n                \"id\": \"urn:oid:2.49.0.1.840.0.52fef07b0c3a98d88109cd1837a99c72cb982c5b.011.2\",\n                \"areaDesc\": \"South Side of Saint Lawrence Island out to 15 NM\",\n                \"geocode\": {\n                    \"SAME\": [\n                        \"058816\"\n                    ],\n                    \"UGC\": [\n                        \"PKZ816\"\n                    ]\n                },\n                \"affectedZones\": [\n                    \"https://api.weather.gov/zones/forecast/PKZ816\"\n                ],\n                \"references\": [],\n                \"sent\": \"2025-12-02T15:49:00-09:00\",\n                \"effective\": \"2025-12-02T15:49:00-09:00\",\n                \"onset\": \"2025-12-02T15:00:00-09:00\",\n                \"expires\": \"2025-12-03T06:00:00-09:00\",\n                \"ends\": \"2025-12-03T17:00:00-09:00\",\n                \"status\": \"Actual\",\n                \"messageType\": \"Alert\",\n                \"category\": \"Met\",\n                \"severity\": \"Severe\",\n                \"certainty\": \"Likely\",\n                \"urgency\": \"Expected\",\n                \"event\": \"Heavy Freezing Spray Warning\",\n                \"sender\": \"w-nws.webmaster@noaa.gov\",\n                \"senderName\": \"NWS Fairbanks AK\",\n                \"headline\": \"Heavy Freezing Spray Warning issued December 2 at 3:49PM AKST until December 3 at 5:00PM AKST by NWS Fairbanks AK\",\n                \"description\": \"Northwestern Alaska Coastal Waters out 100 NM\\n\\nWind forecasts reflect the predominant speed and direction\\nexpected. Sea forecasts represent the average of the highest one-\\nthird of the combined wind-wave and swell height.\\n\\n.TONIGHT...N winds 40 kt. Seas 10 ft. Heavy freezing spray.\\n.WED...N winds 35 kt. Seas 8 ft. Heavy freezing spray.\\n.WED NIGHT...N winds 25 kt. Seas 5 ft. Heavy freezing spray.\\n.THU...NE winds 15 kt. Seas 3 ft. Freezing spray.\\n.THU NIGHT...NE winds 15 kt. Seas 3 ft. Freezing spray.\\n.FRI...NE winds 15 kt. Seas 6 ft. Heavy freezing spray.\\n.FRI NIGHT...NE winds 20 kt. Seas 8 ft. Freezing spray.\\n.SAT...NE winds 25 kt. Seas 10 ft.\\n.SUN...NE winds 35 kt. Seas 10 ft.\",\n                \"instruction\": null,\n                \"response\": \"Avoid\",\n                \"parameters\": {\n                    \"AWIPSidentifier\": [\n                        \"CWFWCZ\"\n                    ],\n                    \"WMOidentifier\": [\n                        \"FZAK52 PAFG 030049\"\n                    ],\n                    \"NWSheadline\": [\n                        \"GALE WARNING IN EFFECT THROUGH WEDNESDAY MORNING... ...HEAVY FREEZING SPRAY WARNING IN EFFECT THROUGH WEDNESDAY AFTERNOON\"\n                    ],\n                    \"BLOCKCHANNEL\": [\n                        \"EAS\",\n                        \"NWEM\",\n                        \"CMAS\"\n                    ],\n                    \"VTEC\": [\n                        \"/O.NEW.PAFG.UP.W.2015.251203T0000Z-251204T0200Z/\"\n                    ],\n                    \"eventEndingTime\": [\n                        \"2025-12-03T17:00:00-09:00\"\n                    ]\n                },\n                \"scope\": \"Public\",\n                \"code\": \"IPAWSv1.0\",\n                \"language\": \"en-US\",\n                \"web\": \"http://www.weather.gov\",\n                \"eventCode\": {\n                    \"SAME\": [\n                        \"NWS\"\n                    ],\n                    \"NationalWeatherService\": [\n                        \"UPW\"\n                    ]\n                }\n            }\n        },\n        {\n            \"id\": \"https://api.weather.gov/alerts/urn:oid:2.49.0.1.840.0.52fef07b0c3a98d88109cd1837a99c72cb982c5b.013.1\",\n            \"type\": \"Feature\",\n            \"geometry\": null,\n            \"properties\": {\n                \"@id\": \"https://api.weather.gov/alerts/urn:oid:2.49.0.1.840.0.52fef07b0c3a98d88109cd1837a99c72cb982c5b.013.1\",\n                \"@type\": \"wx:Alert\",\n                \"id\": \"urn:oid:2.49.0.1.840.0.52fef07b0c3a98d88109cd1837a99c72cb982c5b.013.1\",\n                \"areaDesc\": \"Etolin Strait to Kwemeluk Pass from 15 to 90 NM\",\n                \"geocode\": {\n                    \"SAME\": [\n                        \"058850\"\n                    ],\n                    \"UGC\": [\n                        \"PKZ850\"\n                    ]\n                },\n                \"affectedZones\": [\n                    \"https://api.weather.gov/zones/forecast/PKZ850\"\n                ],\n                \"references\": [],\n                \"sent\": \"2025-12-02T15:49:00-09:00\",\n                \"effective\": \"2025-12-02T15:49:00-09:00\",\n                \"onset\": \"2025-12-02T15:00:00-09:00\",\n                \"expires\": \"2025-12-03T06:00:00-09:00\",\n                \"ends\": \"2025-12-03T17:00:00-09:00\",\n                \"status\": \"Actual\",\n                \"messageType\": \"Alert\",\n                \"category\": \"Met\",\n                \"severity\": \"Moderate\",\n                \"certainty\": \"Likely\",\n                \"urgency\": \"Expected\",\n                \"event\": \"Gale Warning\",\n                \"sender\": \"w-nws.webmaster@noaa.gov\",\n                \"senderName\": \"NWS Fairbanks AK\",\n                \"headline\": \"Gale Warning issued December 2 at 3:49PM AKST until December 3 at 5:00PM AKST by NWS Fairbanks AK\",\n                \"description\": \"Northwestern Alaska Coastal Waters out 100 NM\\n\\nWind forecasts reflect the predominant speed and direction\\nexpected. Sea forecasts represent the average of the highest one-\\nthird of the combined wind-wave and swell height.\\n\\n.TONIGHT...NE winds 40 kt. Seas 12 ft. Blowing snow. Heavy\\nfreezing spray.\\n.WED...NE winds 35 kt. Seas 10 ft. Heavy freezing spray.\\n.WED NIGHT...NE winds 30 kt. Seas 7 ft. Heavy freezing spray.\\n.THU...NE winds 25 kt. Seas 4 ft. Heavy freezing spray.\\n.THU NIGHT...NE winds 20 kt. Seas 4 ft. Heavy freezing spray.\\n.FRI...NE winds 20 kt. Seas 7 ft. Heavy freezing spray.\\n.FRI NIGHT...NE winds 20 kt. Seas 10 ft. Heavy freezing spray.\\n.SAT...NE winds 25 kt. Seas 12 ft.\\n.SUN...NE winds 35 kt. Seas 12 ft.\",\n                \"instruction\": null,\n                \"response\": \"Avoid\",\n                \"parameters\": {\n                    \"AWIPSidentifier\": [\n                        \"CWFWCZ\"\n                    ],\n                    \"WMOidentifier\": [\n                        \"FZAK52 PAFG 030049\"\n                    ],\n                    \"NWSheadline\": [\n                        \"GALE WARNING IN EFFECT THROUGH WEDNESDAY AFTERNOON... ...HEAVY FREEZING SPRAY WARNING IN EFFECT THROUGH WEDNESDAY AFTERNOON\"\n                    ],\n                    \"BLOCKCHANNEL\": [\n                        \"EAS\",\n                        \"NWEM\",\n                        \"CMAS\"\n                    ],\n                    \"VTEC\": [\n                        \"/O.NEW.PAFG.GL.W.2018.251203T0000Z-251204T0200Z/\"\n                    ],\n                    \"eventEndingTime\": [\n                        \"2025-12-03T17:00:00-09:00\"\n                    ]\n                },\n                \"scope\": \"Public\",\n                \"code\": \"IPAWSv1.0\",\n                \"language\": \"en-US\",\n                \"web\": \"http://www.weather.gov\",\n                \"eventCode\": {\n                    \"SAME\": [\n                        \"NWS\"\n                    ],\n                    \"NationalWeatherService\": [\n                        \"GLW\"\n                    ]\n                }\n            }\n        },\n        {\n            \"id\": \"https://api.weather.gov/alerts/urn:oid:2.49.0.1.840.0.52fef07b0c3a98d88109cd1837a99c72cb982c5b.002.1\",\n            \"type\": \"Feature\",\n            \"geometry\": null,\n            \"properties\": {\n                \"@id\": \"https://api.weather.gov/alerts/urn:oid:2.49.0.1.840.0.52fef07b0c3a98d88109cd1837a99c72cb982c5b.002.1\",\n                \"@type\": \"wx:Alert\",\n                \"id\": \"urn:oid:2.49.0.1.840.0.52fef07b0c3a98d88109cd1837a99c72cb982c5b.002.1\",\n                \"areaDesc\": \"Dall Point to Kwikpak Pass out to 15 NM\",\n                \"geocode\": {\n                    \"SAME\": [\n                        \"058802\"\n                    ],\n                    \"UGC\": [\n                        \"PKZ802\"\n                    ]\n                },\n                \"affectedZones\": [\n                    \"https://api.weather.gov/zones/forecast/PKZ802\"\n                ],\n                \"references\": [],\n                \"sent\": \"2025-12-02T15:49:00-09:00\",\n                \"effective\": \"2025-12-02T15:49:00-09:00\",\n                \"onset\": \"2025-12-02T15:00:00-09:00\",\n                \"expires\": \"2025-12-03T06:00:00-09:00\",\n                \"ends\": \"2025-12-03T17:00:00-09:00\",\n                \"status\": \"Actual\",\n                \"messageType\": \"Alert\",\n                \"category\": \"Met\",\n                \"severity\": \"Moderate\",\n                \"certainty\": \"Likely\",\n                \"urgency\": \"Expected\",\n                \"event\": \"Gale Warning\",\n                \"sender\": \"w-nws.webmaster@noaa.gov\",\n                \"senderName\": \"NWS Fairbanks AK\",\n                \"headline\": \"Gale Warning issued December 2 at 3:49PM AKST until December 3 at 5:00PM AKST by NWS Fairbanks AK\",\n                \"description\": \"Northwestern Alaska Coastal Waters out 100 NM\\n\\nWind forecasts reflect the predominant speed and direction\\nexpected. Sea forecasts represent 
